vi "VisionFgvTest.vi"() -> ()   [LabVIEW 2020]
uses:
  builds/VMX_IOB/VMX/VMX_IOB/VMX_IOB.lvlibp/SubVI/System/CamFGV.ctl
  builds/VMX_IOB/VMX/VMX_IOB/VMX_IOB.lvlibp
panel:
  in  "stop":bool
  out "Image":T1(plugin-control)
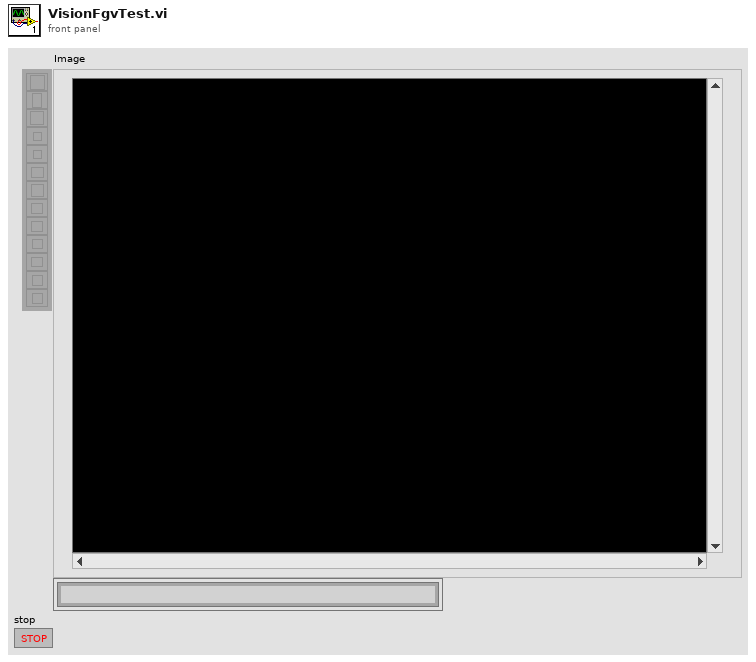
[diagram p1: front panel]
types:
  T1 = typedef "IMAQ Image.ctl" = refnum<image>
  T2 = typedef "VMX_IOB.lvlibp/CamFGV.ctl" = enum16{"Set", "Read", "Close"}
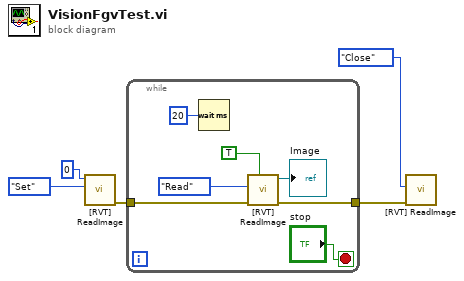
[diagram p0: block diagram]
diagram:
  n1 = call "[RVT] ReadImage.vi"("CamFGV"=CamFGV."Set", "Camera ID"=0) -> ("error out"=w2:errorcluster)  [unwired: 7 in, 2 out]
  n2 = while {
    tunnel: w2 -> [w11]
    tunnel: [w10] -> w1
    stop <- "stop" stop-if-true
    n3 = Wait (ms)(milliseconds to wait=u32 20) -> ()  [unwired: 1 out]
    n4 = call "[RVT] ReadImage.vi"("Continue?"=TRUE, "Error In"=w11, "CamFGV"=CamFGV."Read") -> ("error out"=w10:errorcluster, "Image"=→"Image":T1)  [unwired: 6 in, 1 out]
  }
  n5 = call "[RVT] ReadImage.vi"("Error In"=w1, "CamFGV"=CamFGV."Close") -> ()  [unwired: 7 in, 3 out]
